vi "Read PNA Properties for App.vi"(8 "error in (no error)":errorcluster, 11 "N5222A PNA in":refnum<class "N5222A PNA.lvclass">) -> (0 "error out":errorcluster, 1 "Cal Files by name":string[](array[string]), 3 "N5222A PNA out":refnum<class "N5222A PNA.lvclass">)   [LabVIEW 2018, in "N5222A PNA.lvclass"]
doc: "Read properties from the PNA, for example what cal files are present, so that the main application can be populated with user information."
uses:
  N5222A PNA.lvclass
  N5222A PNA.lvclass/N5222A PNA.ctl
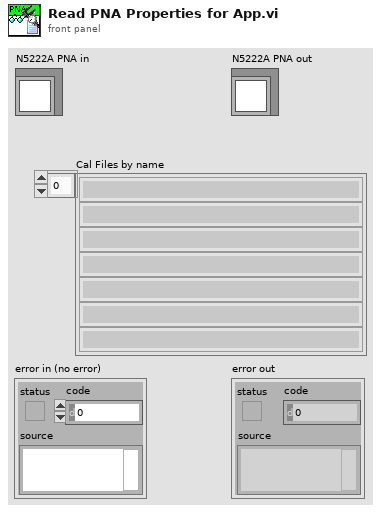
[diagram p1: front panel]
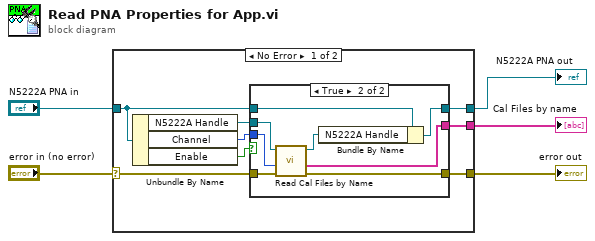
[diagram p0: block diagram]
diagram:
  n1 = case shown="No Error" "error in (no error)" {
    selector: "error in (no error)" -> [w8 w25]
    tunnel: [w7 w25] -> w4
    tunnel: [w10 w24] -> w2
    tunnel: "N5222A PNA in" -> [w11 w24]
    tunnel: [w9 _] -> w1
    frame No Error {
      n2 = Unbundle By Name(w11) -> ("N5222A Handle"=w12:refnum<visa-resource-name>, "Channel"=w13:i32, "Enable"=w6:bool)
      n3 = case shown="True" w6 {
        tunnel: w13 -> [_ w23]
        tunnel: w12 -> [_ w22]
        tunnel: w11 -> [w15 w20]
        tunnel: [w15 w19] -> w10
        tunnel: [_ w18] -> w9
        tunnel: w8 -> [w14 w17]
        tunnel: [w14 w16] -> w7
        frame False {
        }
        frame True {
          n4 = call "Read Cal Files by Name.vi"("Error In (no error)"=w17, "Channel (1)"=w23, "VISA Resource Name"=w22) -> ("error out"=w16:errorcluster, "Cal Files by name"=w18:string[], "VISA Resource Out"=w21:refnum<visa-resource-name>)  [unwired: 6 in]
          n5 = Bundle By Name(cluster=w20, "N5222A Handle"=w21) -> (w19:refnum<class "N5222A PNA.lvclass">)
        }
      }
    }
    frame Error {
    }
  }
  "error out" <- w4
  "N5222A PNA out" <- w2
  "Cal Files by name" <- w1
